vi "Diag. Scale to Corridor.vi"(8 "Command Info In":T2, 10 "Block Inputs":T1, 11 "Starting Position":T5) -> (0 "Command Info Out":T2)   [LabVIEW 2017]
uses:
  <vilib>/Rock Robotics/WPI/Framework/Command Status Info.ctl
  <vilib>/Rock Robotics/WPI/Framework/Completion Status.ctl
  <vilib>/Rock Robotics/WPI/Framework/Completion Notifier.ctl
  Support Code/Starting Position.ctl
  Support Code/Extended Block Inputs.ctl
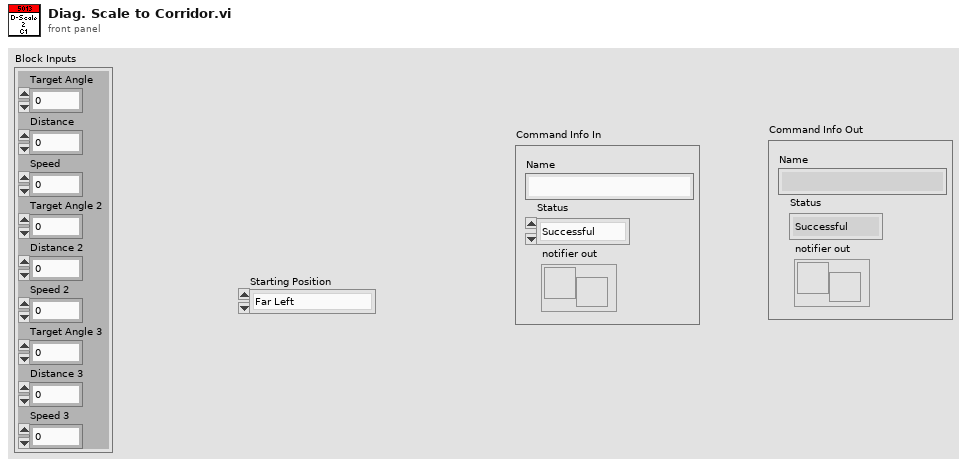
[diagram p1: front panel]
types:
  T1 = typedef "Extended Block Inputs.ctl" = cluster{"Target Angle":dbl, "Distance":dbl, "Speed":dbl, "Target Angle 2":dbl, "Distance 2":dbl, "Speed 2":dbl, "Target Angle 3":dbl, "Distance 3":dbl, "Speed 3":dbl}
  T2 = typedef "Command Status Info.ctl" = cluster{"Name":string, "Status":T3, "notifier out":T4}
  T3 = typedef "Completion Status.ctl" = enum16{"Successful", "Aborted", "Incomplete"}
  T4 = typedef "Completion Notifier.ctl" = refnum<notifier>
  T5 = typedef "Starting Position.ctl" = enum16{"Far Left", "Center", "Far Right"}
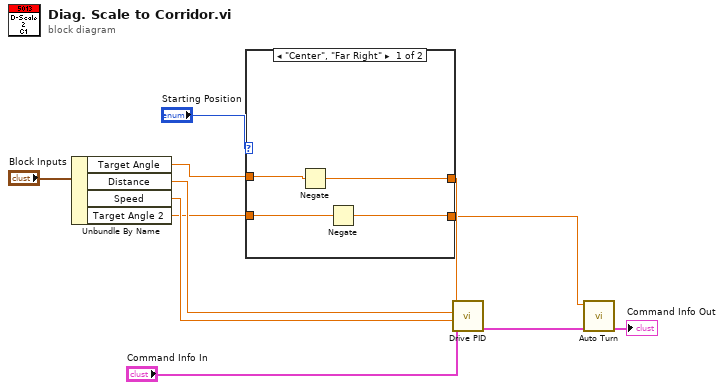
[diagram p0: block diagram]
diagram:
  n1 = Unbundle By Name("Block Inputs") -> ("Target Angle"=w6:dbl, "Distance"=w4:dbl, "Speed"=w3:dbl, "Target Angle 2"=w1:dbl)
  n2 = case shown="\"Center\", \"Far Right\"" "Starting Position" {
    tunnel: w6 -> [w15 w17]
    tunnel: [w14 w17] -> w5
    tunnel: [w12 w16] -> w2
    tunnel: w1 -> [w13 w16]
    frame "Center", "Far Right" {
      n3 = Negate(x=w15) -> (-x=w14:dbl)
      n4 = Negate(x=w13) -> (-x=w12:dbl)
    }
    frame "Far Left", Default {
    }
  }
  n5 = call "Drive PID.vi"("Command Info In"="Command Info In", "Speed"=w3, "Distance"=w4, "Target Angle"=w5) -> ("Command Info Out"=w9:T2)  [unwired: 7 in]
  n6 = call "Auto Turn.vi"("Command Info In"=w9, "Target Angle"=w2) -> ("Command Info Out"=→"Command Info Out":T2)  [unwired: 9 in]
